vi "Read General Page Properties.vi"(8 "error in (no error)":errorcluster, 11 "Page in":refnum<class "Page.lvclass">) -> (0 "error out":errorcluster, 2 "Page Properties":T1, 3 "Page out":refnum<class "Page.lvclass">)   [LabVIEW 2015, in "Page.lvclass"]
uses:
  Page.lvclass
  Custom Device Type Defs/Page Properties.ctl
  XML Controls/Path Cluster.ctl
  XML Controls/help.ctl
  Page.lvclass/Page.ctl
  Configuration Tool.lvlib
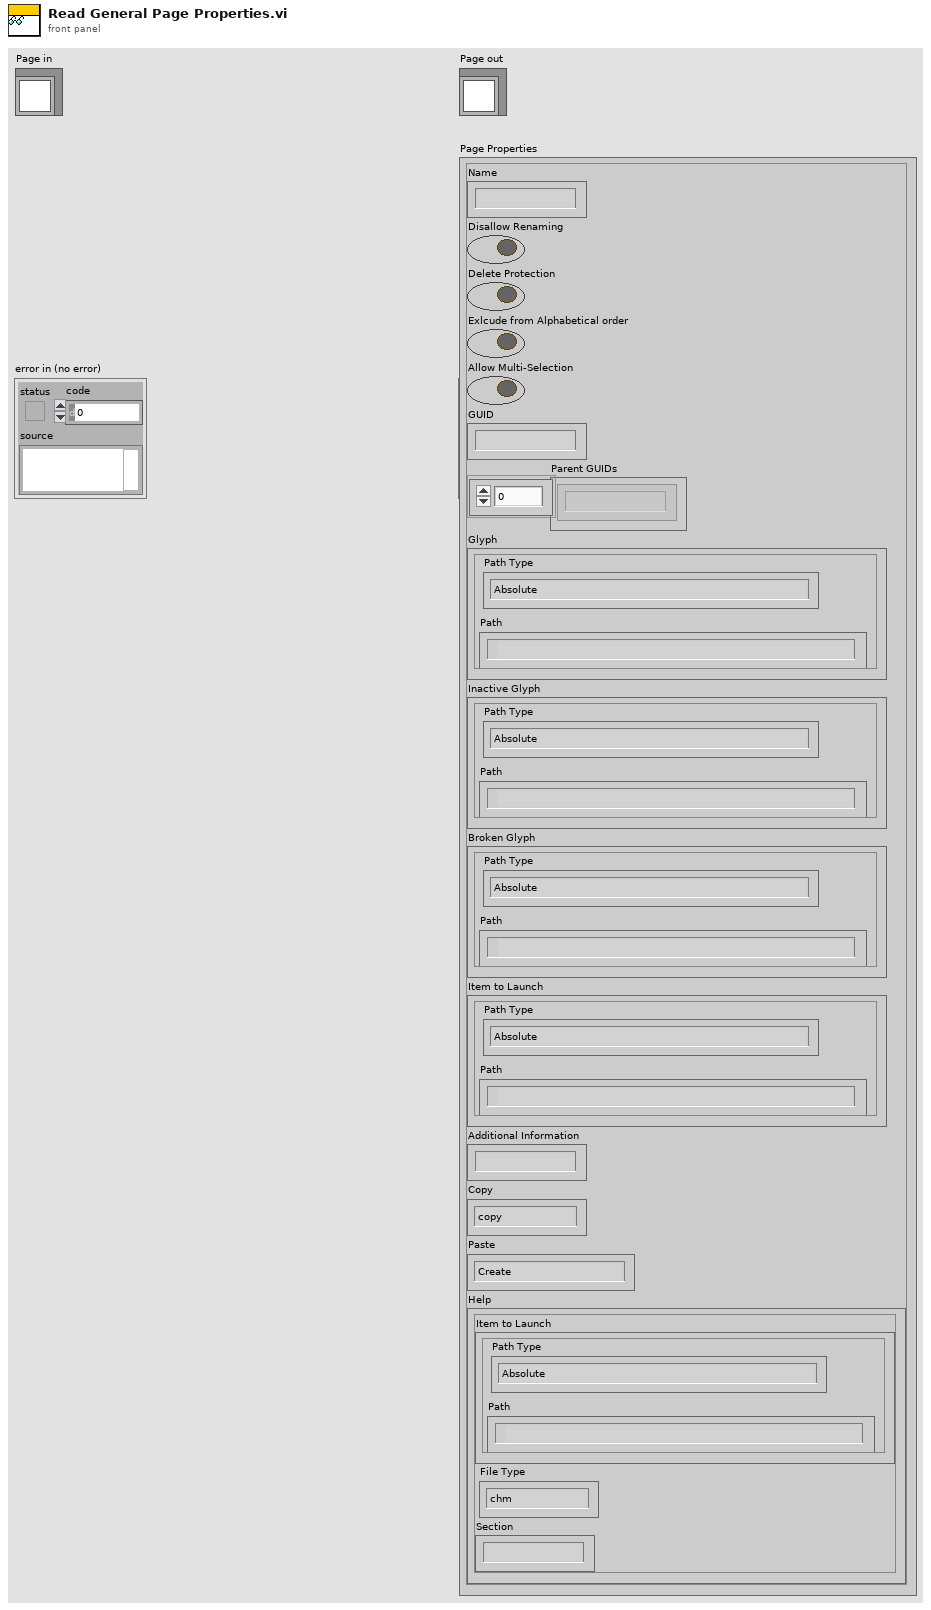
[diagram p1: front panel]
types:
  T1 = typedef "Page Properties.ctl" = cluster{"Name":string, "Disallow Renaming":bool, "Delete Protection":bool, "Exlcude from Alphabetical order":bool, "Allow Multi-Selection":bool, "GUID":string, "Parent GUIDs":string[], "Glyph":T2, "Inactive Glyph":T2, "Broken Glyph":T2, "Item to Launch":T2, "Additional Information":string, "Copy":enum16{"copy", "disabled"}, "Paste":enum16{"Create", "CreatIfNotExists_GUID", "CreatIfNotExists_Name", "Replace", "Dialog"}, "Help":T3}
  T2 = typedef "Configuration Tool.lvlib/Path Cluster.ctl" = cluster{"Path":path, "Path Type":enum16{"Absolute", "To Base", "To Common Doc Dir", "To Application Data Dir"}}
  T3 = typedef "Configuration Tool.lvlib/help.ctl" = cluster{"Item to Launch":T2, "Section":string, "File Type":enum16{"chm", "other"}}
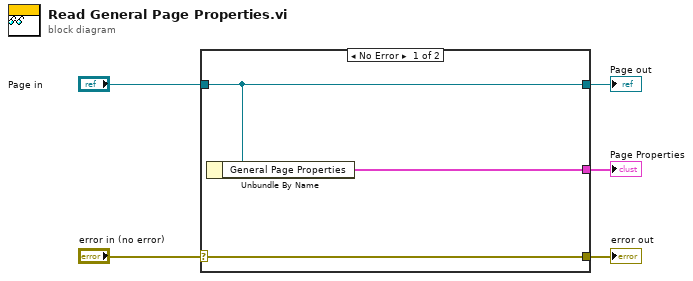
[diagram p0: block diagram]
diagram:
  n1 = case shown="No Error" "error in (no error)" {
    selector: "error in (no error)" -> [w8 w9]
    tunnel: [w8 w9] -> w4
    tunnel: [w7 w10] -> w2
    tunnel: "Page in" -> [w7 w10]
    tunnel: [w6 _] -> w1
    frame No Error {
      n2 = Unbundle By Name(w7) -> ("General Page Properties"=w6:T1)
    }
    frame Error {
    }
  }
  "error out" <- w4
  "Page out" <- w2
  "Page Properties" <- w1
